vi "init control_ring.vi"(10 "Ring Refnum":refnum<vi>) -> (2 "Control out":refnum<class "Control.lvclass">)   [LabVIEW 2010, in "Control.lvclass"]
uses:
  Control.lvclass
  Ring Control/Ring Control.lvclass
  Control.lvclass/Control.ctl
panel:
  in  "Control in":refnum<class "Control.lvclass">
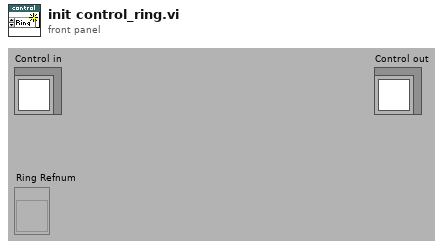
[diagram p1: front panel]
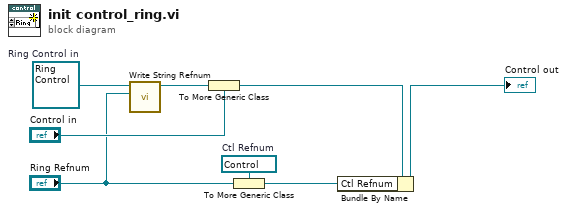
[diagram p0: block diagram]
diagram:
  w1 = refnum<class "Ring Control.lvclass"> refnum  # Ring Control in
  w5 = refnum<vi> refnum  # Ctl Refnum
  n1 = call "Write String Refnum.vi"("Ring Refnum"="Ring Refnum", "Ring Control in"=w1) -> ("Ring Control out"=w3:refnum<class "Ring Control.lvclass">)  [unwired: 8 in, 1 out]
  n2 = To More Generic Class(target class="Control in", reference=w3) -> (generic class reference=w4:refnum<class "Control.lvclass">)
  n3 = To More Generic Class(target class=w5, reference="Ring Refnum") -> (generic class reference=w6:refnum<vi>)
  n4 = Bundle By Name(cluster=w4, "Ctl Refnum"=w6) -> (→"Control out":refnum<class "Control.lvclass">)
